vi "From Serial Form.vi"(6 "Serial Version":T1, 10 "Deserializer in":refnum<class "Deserializer.lvclass">, 11 "PAS Cell Data in":refnum<class "PAS Cell Data.lvclass">) -> (0 "error out":errorcluster, 2 "Deserializer out":refnum<class "Deserializer.lvclass">, 3 "PAS Cell Data out":refnum<class "PAS Cell Data.lvclass">)   [LabVIEW 2014, in "PAS Cell Data.lvclass"]
uses:
  PAS Cell Data.lvclass
  <vilib>/NI/AQ Character Lineator/Deserializer/Deserializer.lvclass
  <vilib>/NI/AQ Character Lineator/Serialization Common/Serial Version.ctl
  <vilib>/NI/AQ Character Lineator/Serializable/Remove Double.vi
  <vilib>/NI/AQ Character Lineator/Serializable/Remove Double Array.vi
  <vilib>/Analysis/Matrix/Numeric/Conversions/Array To Matrix - RA2.vi
  Data/Data.lvclass
  <vilib>/NI/AQ Character Lineator/Serializable/Serializable.lvclass
  <vilib>/Analysis/Matrix/NI_Matrix.lvlib
  <vilib>/NI/AQ Character Lineator/Serializable Analog Waveform/Serializable Analog Waveform.lvclass
  <vilib>/NI/AQ Character Lineator/Serialization Common/Serialization Common.lvlib
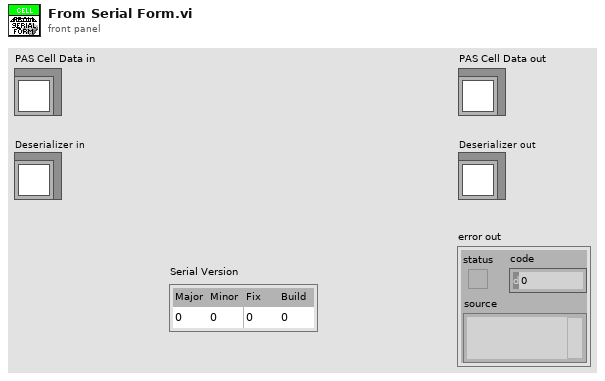
[diagram p1: front panel]
types:
  T1 = typedef "Serialization Common.lvlib/Serial Version.ctl" = cluster{"Major":u16, "Minor":u16, "Fix":u16, "Build":u16}
  T2 = typedef "NI_Matrix.lvlib/RealMatrix.ctl" = dbl[][]
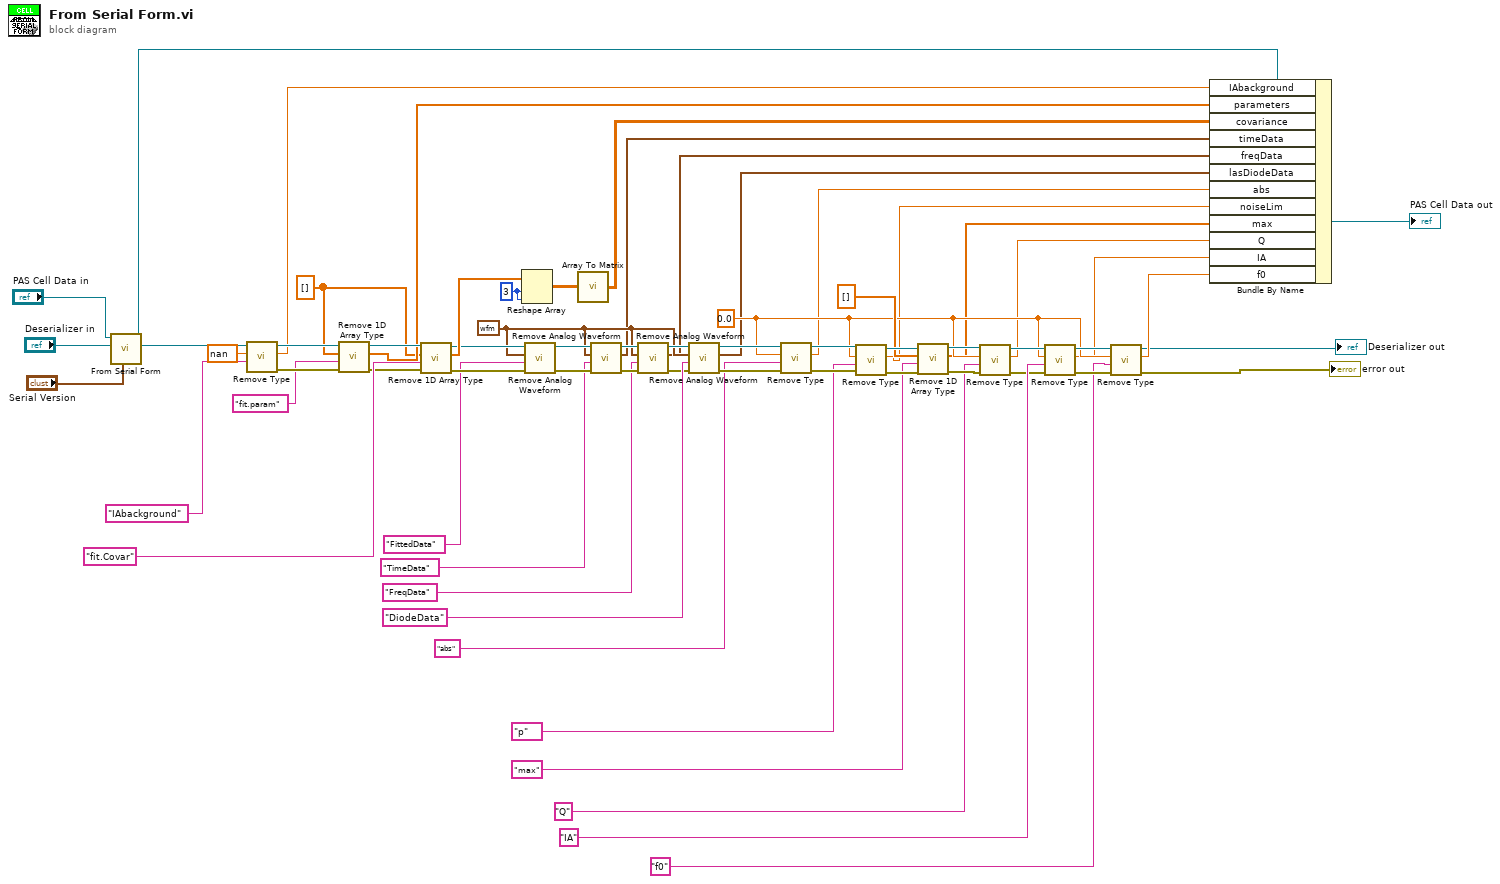
[diagram p0: block diagram]
diagram:
  w2 = dbl[] [] ("Default Value")
  w23 = 0.0 ("Default Value")
  w44 = waveform(dbl) {"t0"=timestamp(0 s since 1904-01-01), "dt"=1.0, "Y"=[]} ("Default Value")
  w56 = 3 ("dimension size")
  n1 = call-parent "From Serial Form.vi"("Serial Version"="Serial Version", "Deserializer in"="Deserializer in", "Data in"="PAS Cell Data in") -> ("Deserializer out"=w61:refnum<class "Deserializer.lvclass">, "Data out"=w22:refnum<class "PAS Cell Data.lvclass">)  [unwired: 6 in, 1 out]
  "PAS Cell Data out" <- w22
  n2 = call-poly <vilib>:"Remove Type.vi"("Name"="IAbackground", "Default Value"=nan, "Deserializer in"=w61) -> ("error out"=w9:errorcluster, "Numeric"=w5:dbl, "Deserializer out"=w10:refnum<class "Deserializer.lvclass">)  [unwired: 5 in, 1 out]
  n3 = call-poly <vilib>:"Remove 1D Array Type.vi"("error in (no error)"=w9, "Name"="fit.param", "Default Value"=w2, "Deserializer in"=w10) -> ("error out"=w7:errorcluster, "Doubles"=w6:dbl[], "Deserializer out"=w8:refnum<class "Deserializer.lvclass">)  [unwired: 4 in, 1 out]
  n4 = call-poly <vilib>:"Remove 1D Array Type.vi"("error in (no error)"=w7, "Name"="fit.Covar", "Default Value"=w2, "Deserializer in"=w8) -> ("error out"=w53:errorcluster, "Doubles"=w57:dbl[], "Deserializer out"=w54:refnum<class "Deserializer.lvclass">)  [unwired: 4 in, 1 out]
  n5 = Reshape Array(w57, w56, w56) -> (w55:dbl[][])
  n6 = call <vilib>:"Remove Analog Waveform.vi"("error in (no error)"=w53, "Name"="FittedData", "Default Value"=w44, "Deserializer in"=w54) -> ("error out"=w50:errorcluster, "Deserializer out"=w51:refnum<class "Deserializer.lvclass">)  [unwired: 4 in, 2 out]
  n7 = call-poly <vilib>:"Array To Matrix.vi"("Real 2D Array"=w55) -> ("Real Matrix"=w11:T2)
  n8 = call <vilib>:"Remove Analog Waveform.vi"("error in (no error)"=w50, "Name"="TimeData", "Default Value"=w44, "Deserializer in"=w51) -> ("error out"=w47:errorcluster, "Analog Waveform"=w12:waveform(dbl), "Deserializer out"=w48:refnum<class "Deserializer.lvclass">)  [unwired: 4 in, 1 out]
  n9 = call <vilib>:"Remove Analog Waveform.vi"("error in (no error)"=w47, "Name"="FreqData", "Default Value"=w44, "Deserializer in"=w48) -> ("error out"=w13:errorcluster, "Analog Waveform"=w14:waveform(dbl), "Deserializer out"=w45:refnum<class "Deserializer.lvclass">)  [unwired: 4 in, 1 out]
  n10 = call <vilib>:"Remove Analog Waveform.vi"("error in (no error)"=w13, "Name"="DiodeData", "Default Value"=w44, "Deserializer in"=w45) -> ("error out"=w41:errorcluster, "Analog Waveform"=w15:waveform(dbl), "Deserializer out"=w42:refnum<class "Deserializer.lvclass">)  [unwired: 4 in, 1 out]
  n11 = call-poly <vilib>:"Remove Type.vi"("error in (no error)"=w41, "Name"="abs", "Default Value"=w23, "Deserializer in"=w42) -> ("error out"=w38:errorcluster, "Numeric"=w16:dbl, "Deserializer out"=w39:refnum<class "Deserializer.lvclass">)  [unwired: 4 in, 1 out]
  n12 = call-poly <vilib>:"Remove Type.vi"("error in (no error)"=w38, "Name"="p", "Default Value"=w23, "Deserializer in"=w39) -> ("error out"=w35:errorcluster, "Numeric"=w17:dbl, "Deserializer out"=w36:refnum<class "Deserializer.lvclass">)  [unwired: 4 in, 1 out]
  n13 = call-poly <vilib>:"Remove 1D Array Type.vi"("error in (no error)"=w35, "Name"="max", "Default Value"=dbl[] [], "Deserializer in"=w36) -> ("error out"=w31:errorcluster, "Doubles"=w18:dbl[], "Deserializer out"=w32:refnum<class "Deserializer.lvclass">)  [unwired: 4 in, 1 out]
  n14 = call-poly <vilib>:"Remove Type.vi"("error in (no error)"=w31, "Name"="Q", "Default Value"=w23, "Deserializer in"=w32) -> ("error out"=w27:errorcluster, "Numeric"=w19:dbl, "Deserializer out"=w29:refnum<class "Deserializer.lvclass">)  [unwired: 4 in, 1 out]
  n15 = call-poly <vilib>:"Remove Type.vi"("error in (no error)"=w27, "Name"="IA", "Default Value"=w23, "Deserializer in"=w29) -> ("error out"=w25:errorcluster, "Numeric"=w20:dbl, "Deserializer out"=w26:refnum<class "Deserializer.lvclass">)  [unwired: 4 in, 1 out]
  n16 = call-poly <vilib>:"Remove Type.vi"("error in (no error)"=w25, "Name"="f0", "Default Value"=w23, "Deserializer in"=w26) -> ("error out"=→"error out":errorcluster, "Numeric"=w21:dbl, "Deserializer out"=→"Deserializer out":refnum<class "Deserializer.lvclass">)  [unwired: 4 in, 1 out]
  n17 = Bundle By Name(cluster=w22, "IAbackground"=w5, "parameters"=w6, "covariance"=w11, "timeData"=w12, "freqData"=w14, "lasDiodeData"=w15, "abs"=w16, "noiseLim"=w17, "max"=w18, "Q"=w19, "IA"=w20, "f0"=w21) -> ()  [unwired: 1 out]
